vi "Allocate Arrays.vi"(8 "error in (no error)":errorcluster, 11 "PXI in":refnum<class "PXI.lvclass">) -> (0 "error out":errorcluster, 3 "PXI out":refnum<class "PXI.lvclass">)   [LabVIEW 2013, in "PXI.lvclass"]
uses:
  PXI.lvclass
  PXI.lvclass/PXI.ctl
  <resource>/objmgr/daqmx.rc
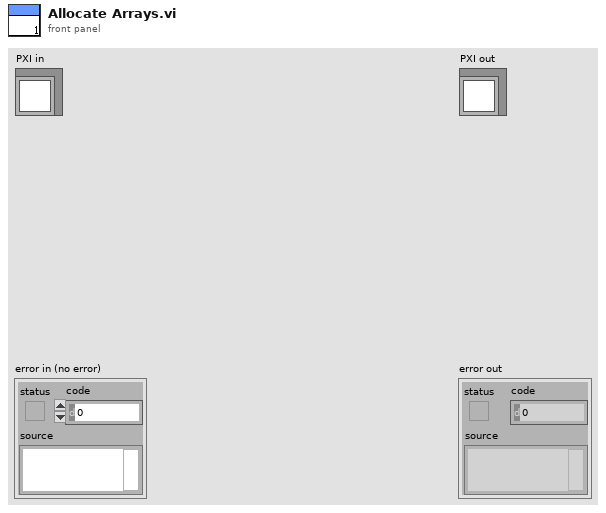
[diagram p1: front panel]
types:
  T1 = typedef "Task Definition.ctl" = cluster{"task_type":T2, "names":string[], "physical channels":tag, "min_value":dbl, "max_value":dbl, "task_number":i32}
  T2 = typedef "Task Types.ctl" = enum16{"Analog Input", "Analog Output", "Digital Input", "Digital Output"}
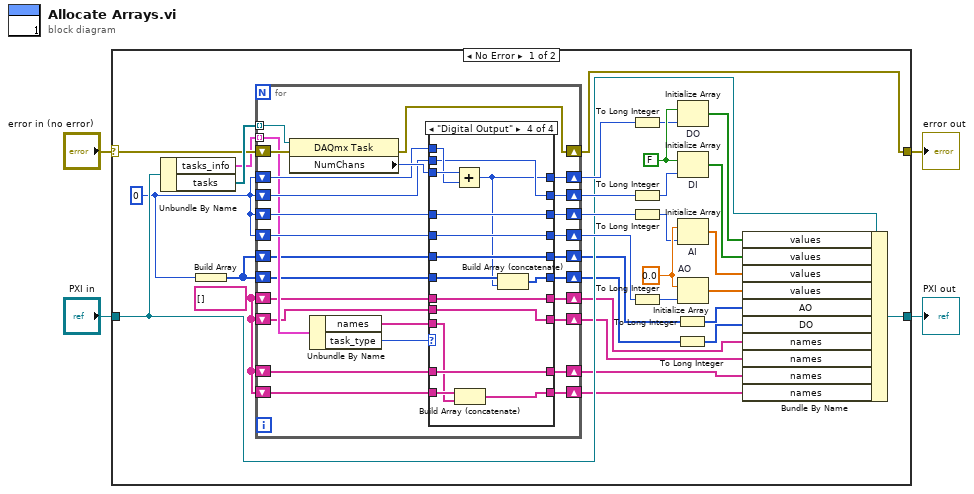
[diagram p0: block diagram]
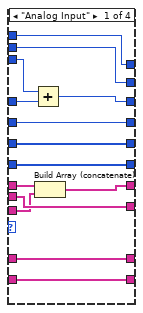
[diagram p2: hidden frame]
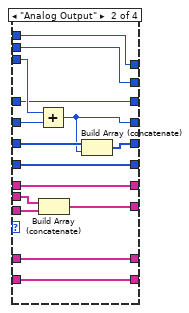
[diagram p3: hidden frame]
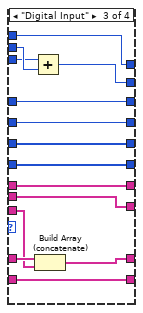
[diagram p4: hidden frame]
diagram:
  n1 = case shown="No Error" "error in (no error)" {
    selector: "error in (no error)" -> [w34 w122]
    tunnel: [w26 w122] -> w3
    tunnel: [w24 w121] -> w1
    tunnel: "PXI in" -> [w25 w121]
    frame No Error {
      w5 = string[] []
      w13 = u32 0 ("NumChans")
      w32 = FALSE
      w33 = 0.0 ("element")
      n2 = Unbundle By Name(w25) -> ("tasks_info"=w19:T1[], "tasks"=w35:refnum<k21>[])
      n3 = Build Array(w13) -> (w11:u32[])
      n4 = for {
        tunnel: w19 -> [w52] mode=indexing
        tunnel: w35 -> [w62] mode=indexing
        shift-right: [w60] -> w26
        shift-left: w34 -> [w61]
        shift-right: [w50] -> w30
        shift-left: w13 -> [w59]
        shift-right: [w48] -> w29
        shift-left: w13 -> [w57]
        shift-right: [w49] -> w28
        shift-left: w13 -> [w55]
        shift-right: [w51] -> w27
        shift-left: w13 -> [w56]
        shift-right: [w46] -> w12
        shift-left: w11 -> [w47]
        shift-right: [w44] -> w10
        shift-left: w11 -> [w45]
        shift-right: [w43] -> w7
        shift-left: w5 -> [w42]
        shift-right: [w41] -> w6
        shift-left: w5 -> [w40]
        shift-right: [w39] -> w8
        shift-left: w5 -> [w38]
        shift-right: [w37] -> w9
        shift-left: w5 -> [w36]
        n5 = property class="DAQmx Task"(reference=w62, error in=w61) -> (error out=w60:errorcluster, "NumChans"=w58:u32)  [unwired: 1 out]
        n6 = Unbundle By Name(w52) -> ("names"=w53:string[], "task_type"=w54:T2)
        n7 = case shown="\"Digital Output\"" w54 {
          tunnel: w59 -> [w75 w90 w100 w116]
          tunnel: w58 -> [w74 w91 w103 w120]
          tunnel: [w76 w90 w100 w116] -> w50
          tunnel: w57 -> [w71 w87 w101 w117]
          tunnel: [w71 w83 w101 w117] -> w48
          tunnel: w56 -> [w72 w89 w104 w118]
          tunnel: [w72 w89 w105 w118] -> w51
          tunnel: [w73 w88 w102 w112] -> w49
          tunnel: w55 -> [w73 w88 w102 w119]
          tunnel: w53 -> [w65 w80 w93 w106]
          tunnel: w47 -> [w70 w84 w99 w115]
          tunnel: [w70 w86 w99 w115] -> w46
          tunnel: w45 -> [w69 w85 w98 w113]
          tunnel: [w69 w85 w98 w114] -> w44
          tunnel: [w68 w82 w97 w111] -> w43
          tunnel: w42 -> [w68 w81 w97 w111]
          tunnel: [w67 w79 w96 w110] -> w41
          tunnel: w40 -> [w66 w79 w96 w110]
          tunnel: [w64 w78 w95 w109] -> w39
          tunnel: w38 -> [w64 w78 w94 w109]
          tunnel: [w63 w77 w92 w108] -> w37
          tunnel: w36 -> [w63 w77 w92 w107]
          frame "Analog Input" {
            n8 = Add(x=w74, y=w75) -> (x+y=w76:u32)
            n9 = Build Array (concatenate)(w66, w65) -> (w67:string[])
          }
          frame "Analog Output" {
            n10 = Add(x=w91, y=w87) -> (x+y=w83:u32)
            n11 = Build Array (concatenate)(w81, w80) -> (w82:string[])
            n12 = Build Array (concatenate)(w84, w83) -> (w86:u32[])
          }
          frame "Digital Input" {
            n13 = Add(x=w103, y=w104) -> (x+y=w105:u32)
            n14 = Build Array (concatenate)(w94, w93) -> (w95:string[])
          }
          frame "Digital Output" {
            n15 = Add(x=w120, y=w119) -> (x+y=w112:u32)
            n16 = Build Array (concatenate)(w107, w106) -> (w108:string[])
            n17 = Build Array (concatenate)(w113, w112) -> (w114:u32[])
          }
        }
      }
      n18 = To Long Integer(number=w28) -> (32bit integer=w31:i32)
      n19 = To Long Integer(number=w27) -> (32bit integer=w16:i32)
      n20 = To Long Integer(number=w30) -> (32bit integer=w15:i32)
      n21 = To Long Integer(number=w29) -> (32bit integer=w17:i32)
      n22 = To Long Integer(number=w12) -> (32bit integer=w18:i32[])
      n23 = To Long Integer(number=w10) -> (32bit integer=w14:i32[])
      n24 = Initialize Array "DO"(w32, w31) -> (w23:bool[])
      n25 = Initialize Array "DI"(w32, w16) -> (w22:bool[])
      n26 = Initialize Array "AI"(w33, w15) -> (w21:dbl[])
      n27 = Initialize Array "AO"(w33, w17) -> (w20:dbl[])
      n28 = Bundle By Name(cluster=w25, "values"=w23, "values"=w22, "values"=w21, "values"=w20, "AO"=w18, "DO"=w14, "names"=w6, "names"=w7, "names"=w8, "names"=w9) -> (w24:refnum<class "PXI.lvclass">)
    }
    frame Error {
    }
  }
  "error out" <- w3
  "PXI out" <- w1
